vi "arduinoTemps.vi"() -> ()   [LabVIEW 2024]
uses:
  <vilib>/Instr/_visa.llb/VISA Configure Serial Port (Instr).vi
panel:
  in  "Stop":bool
  out "Direct Output":string
  out "temp4":dbl
  out "temp3":dbl
  out "temp2":dbl
  out "temp1":dbl
  out "error out":errorcluster
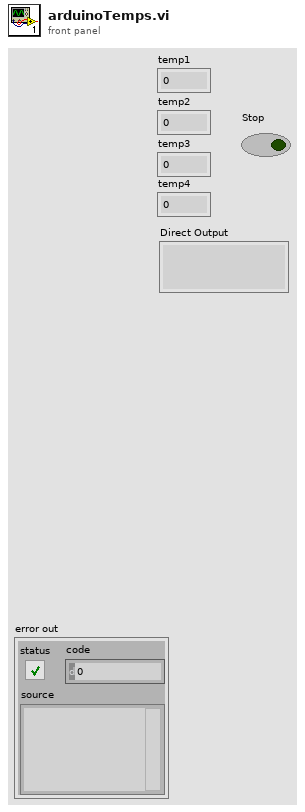
[diagram p1: front panel]
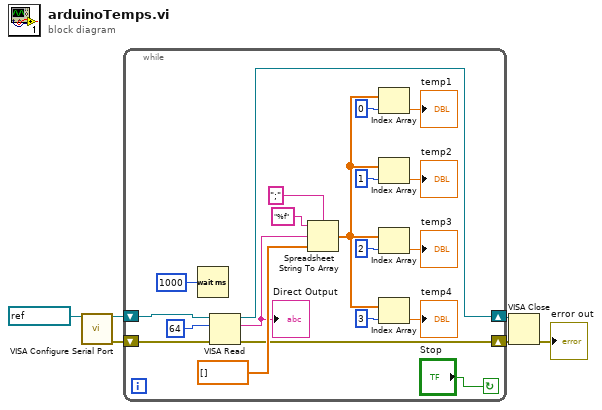
[diagram p0: block diagram]
diagram:
  n1 = call-poly "VISA Configure Serial Port"("VISA resource name"=refnum<visa-resource-name> "COM5") -> ("VISA resource name out"=w5:refnum<visa-resource-name>, "error out"=w4:errorcluster)  [unwired: 13 in]
  n2 = while {
    shift-right: [w11] -> w3
    shift-left: w5 -> [w13]
    shift-right: [w10] -> w2
    shift-left: w4 -> [w12]
    stop <- "Stop" continue-if-true
    n3 = Wait (ms)(milliseconds to wait=u32 1000) -> ()  [unwired: 1 out]
    n4 = VISA Read(VISA resource name=w13, byte count=u32 64, error in (no error)=w12) -> (VISA resource name out=w11:refnum<visa-resource-name>, read buffer=w9:string, error out=w10:errorcluster)  [unwired: 1 out]
    "Direct Output" <- w9
    n5 = Spreadsheet String To Array(delimiter (Tab)=";", format string="%f", spreadsheet string=w9, array type (2D Dbl)=dbl[] []) -> (array=w15:dbl[])
    n6 = Index Array(array=w15, index=0) -> (element=→"temp1":dbl)
    n7 = Index Array(array=w15, index=1) -> (element=→"temp2":dbl)
    n8 = Index Array(array=w15, index=2) -> (element=→"temp3":dbl)
    n9 = Index Array(array=w15, index=3) -> (element=→"temp4":dbl)
  }
  n10 = VISA Close(VISA resource name=w3, error in (no error)=w2) -> (error out=→"error out":errorcluster)
